vi "Configure Averaging.vi"(5 "Enable Step Detection (T: Enable)":bool=TRUE, 6 "Auto Averaging (T: Enable)":bool=TRUE, 7 "Enable Averaging (T: Enable)":bool=TRUE, 8 "error in (no error)":errorcluster, 9 "Averaging Count (4)":i32=4, 10 "Averaging Buffer Size (1)":i32=1, 11 "VISA resource name":refnum<visa-resource-name>) -> (0 "error out":errorcluster, 3 "VISA resource name out":refnum<visa-resource-name>)   [LabVIEW 2014, in "Agilent U2000 Series.lvlib"]
doc: "Controls the settings which dictate how the average of the measurement is calculated."
uses:
  Agilent U2000 Series.lvlib
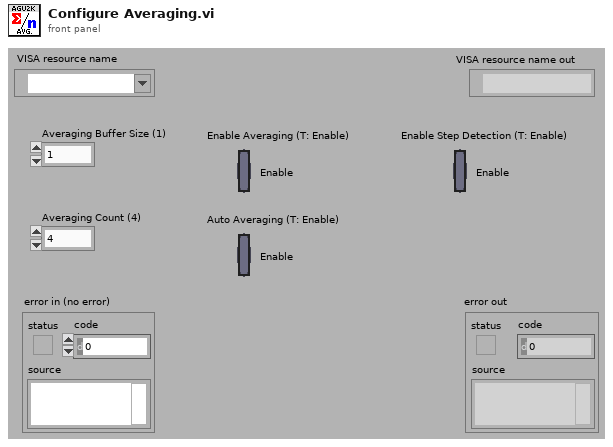
[diagram p1: front panel]
types:
  T1 = typedef "Agilent U2000 Series.lvlib/Extended User Data.ctl" = cluster{"U2000 Series Mode":u16, "Trigger Source Int/Ext":bool}
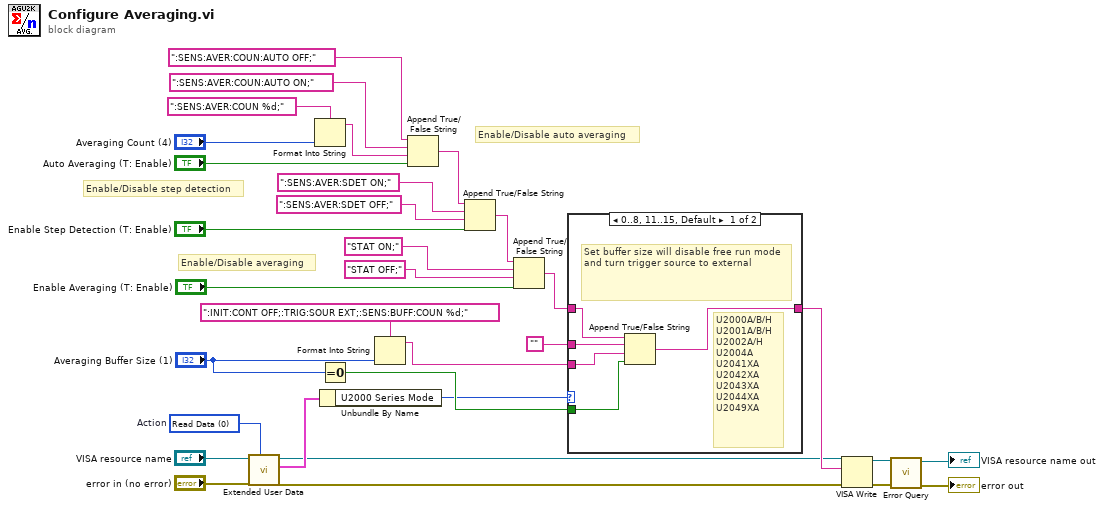
[diagram p0: block diagram]
diagram:
  w2 = 0 items=["Read Data", "Write Data", "Clear Data", "Clear ALL Data"]  # Action
  # "Enable/Disable averaging"
  # "Enable/Disable step detection"
  # "Enable/Disable auto averaging"
  n1 = call "Extended User Data.vi"("Action (1: Write Data)"=w2, "error in (no error)"="error in (no error)", "VISA resource name"="VISA resource name") -> ("error out"=w4:errorcluster, "User Data Out"=w7:T1, "VISA resource name out"=w1:refnum<visa-resource-name>)  [unwired: 1 in, 5 out]
  n2 = Format Into String(format string=":SENS:AVER:COUN %d;", "Averaging Count (4)") -> (resulting string=w21:string)  [unwired: 2 in, 1 out]
  n3 = Equal To 0?(x="Averaging Buffer Size (1)") -> (x = 0?=w10:bool)
  n4 = Unbundle By Name(w7) -> ("U2000 Series Mode"=w3:u16)
  n5 = Format Into String(format string=":INIT:CONT OFF;:TRIG:SOUR EXT;:SENS:BUFF:COUN %d;", "Averaging Buffer Size (1)") -> (resulting string=w9:string)  [unwired: 2 in, 1 out]
  n6 = Append True/False String(1:"Auto Averaging (T: Enable)", 2:w21, 3:":SENS:AVER:COUN:AUTO ON;", 4:":SENS:AVER:COUN:AUTO OFF;") -> (0:w19:string)
  n7 = Append True/False String(1:"Enable Step Detection (T: Enable)", 2:":SENS:AVER:SDET OFF;", 3:":SENS:AVER:SDET ON;", 4:w19) -> (0:w18:string)
  n8 = Append True/False String(1:"Enable Averaging (T: Enable)", 2:"STAT OFF;", 3:"STAT ON;", 4:w18) -> (0:w12:string)
  n9 = case shown="0..8, 11..15, Default" w3 {
    tunnel: w12 -> [w34 w38]
    tunnel: [w33 w38] -> w11
    tunnel: w10 -> [w37 _]
    tunnel: w9 -> [w36 _]
    tunnel: "" -> [w35 _]
    frame 0..8, 11..15, Default {
      # "U2000A/B/H\nU2001A/B/H\nU2002A/H\nU2004A\nU2041XA\nU2042XA\nU2043XA\nU2044XA\nU2049XA"
      # "Set buffer size will disable free run mode and turn trigger source to external"
      n10 = Append True/False String(1:w37, 2:w36, 3:w35, 4:w34) -> (0:w33:string)
    }
    frame 9, 10 {
      # "U2021XA\nU2022XA"
    }
  }
  n11 = VISA Write(VISA resource name=w1, write buffer=w11, error in (no error)=w4) -> (VISA resource name out=w16:refnum<visa-resource-name>, error out=w15:errorcluster)  [unwired: 1 out]
  n12 = call "Error Query.vi"("error in (no error)"=w15, "VISA resource name"=w16) -> ("error out"=→"error out":errorcluster, "VISA resource name out"=→"VISA resource name out":refnum<visa-resource-name>)  [unwired: 8 out]
